vi "Basic Example.vi"() -> ()   [LabVIEW 2014]
uses:
  <userlib>/_NI SPI IP/FPGA/Controllers/Public/Transfer Settings.ctl
  vi.lib/SPIAPI/Controls/SPI Settings.ctl
  vi.lib/SPIAPI/Controls/Signal Properties.ctl
  <vilib>/rvi/Emulation/niFpgaGetClockAttributes.vi
  <vilib>/rvi/Emulation/niFpgaSctlEmulationGetInTimedLoop.vi
  <vilib>/rvi/Emulation/niFpgaEmulationReportErrorSimple.vi
  <vilib>/rvi/interface/RandomDataEmulation/niFpgaRandomDataHandleErrors.vi
  <vilib>/rvi/Emulation/niFpgaCriticalErrorInLSC.vi
  <vilib>/rvi/DataTransferAndStorage/Container/XNode/niFpgaContainer.xnode
  <vilib>/rvi/interface/RandomDataEmulation/nirviRandomDataFpgaReadWriteTemplate.vi
  <userlib>/_NI SPI IP/FPGA/Controllers/NI SPI IP FPGA.lvlib
panel:
  in  "data rate (S/s)":u32=10000
  in  "Chip Select":u8
  in  "SPI Command":u64
  in  "SPI PHY Settings":T1 {"Direction Change Bit" max=64 step=1; "Transfer Length (bits)" min=1 max=64 step=1}
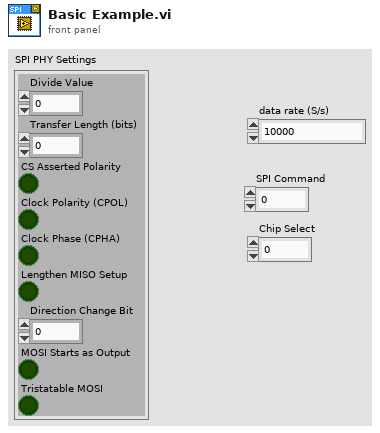
[diagram p1: front panel]
types:
  T1 = typedef "NI SPI IP FPGA.lvlib/Transfer Settings.ctl" = cluster{"Divide Value":u8, "Transfer Length (bits)":u8, "CS Asserted Polarity":bool, "Clock Polarity (CPOL)":bool, "Clock Phase (CPHA)":bool, "Lengthen MISO Setup":bool, "Direction Change Bit":u8, "MOSI Starts as Output":bool, "Tristatable MOSI":bool}
  T2 = typedef "SPI Settings.ctl" = cluster{"SCLK":T3, "Signal Settings":cluster{"MISO":refnum<k21>, "Signal_Enable":refnum<k21>, "Output?":bool}, "MOSI":T3, "CS0":T3, "CS1":T3, "CS2":T3, "CS3":T3, "CS4":T3, "CS5":T3}
  T3 = typedef "Signal Properties.ctl" = cluster{"Signal":refnum<k21>, "Signal_Enable":refnum<k21>, "Output?":bool}
  T4 = typedef "All SPI Settings.ctl" = cluster{"SPI Signal Settings":T2, "SPI Internal Signals":T5, "SPI PHY Settings":T1, "SPI Engine Source":refnum<k21>}
  T5 = typedef "Internal Data (SPI API).ctl" = cluster{"DLU To SPI Engine Data FIFO":refnum<k21>, "SPI Engine to DLU Data FIFO":refnum<k21>, "Data to SPI Engine (Cache) Register":refnum<k21>, "SPI PHY Settings to SPI Engine (Cahche) Register":refnum<k21>}
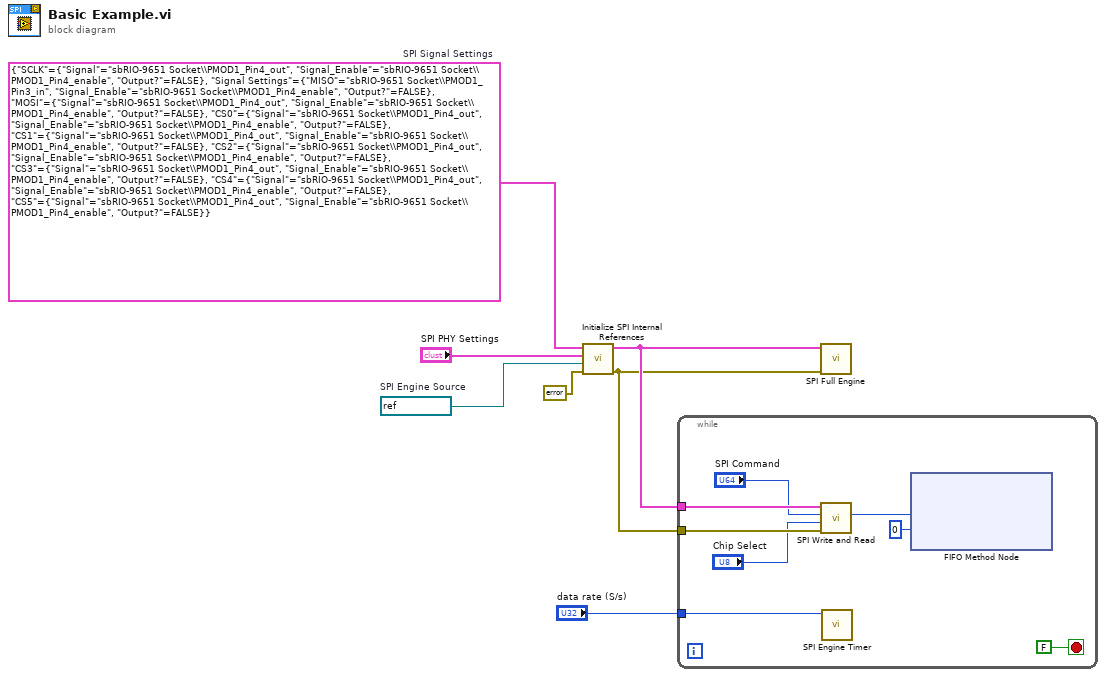
[diagram p0: block diagram]
diagram:
  w7 = T2 {"SCLK"={"Signal"="sbRIO-9651 Socket\\PMOD1_Pin4_out", "Signal_Enable"="sbRIO-9651 Socket\\PMOD1_Pin4_enable", "Output?"=FALSE}, "Signal Settings"={"MISO"="sbRIO-9651 Socket\\PMOD1_Pin3_in", "Signal_Enable"="sbRIO-9651 Socket\\PMOD1_Pin4_enable", "Output?"=FALSE}, "MOSI"={"Signal"="sbRIO-9651 Socket\\PMOD1_Pin4_out", "Signal_Enable"="sbRIO-9651 Socket\\PMOD1_Pin4_enable", "Output?"=FALSE}, "CS0"={"Signal"="sbRIO-9651 Socket\\PMOD1_Pin4_out", "Signal_Enable"="sbRIO-9651 Socket\\PMOD1_Pin4_enable", "Output?"=FALSE}, "CS1"={"Signal"="sbRIO-9651 Socket\\PMOD1_Pin4_out", "Signal_Enable"="sbRIO-9651 Socket\\PMOD1_Pin4_enable", "Output?"=FALSE}, "CS2"={"Signal"="sbRIO-9651 Socket\\PMOD1_Pin4_out", "Signal_Enable"="sbRIO-9651 Socket\\PMOD1_Pin4_enable", "Output?"=FALSE}, "CS3"={"Signal"="sbRIO-9651 Socket\\PMOD1_Pin4_out", "Signal_Enable"="sbRIO-9651 Socket\\PMOD1_Pin4_enable", "Output?"=FALSE}, "CS4"={"Signal"="sbRIO-9651 Socket\\PMOD1_Pin4_out", "Signal_Enable"="sbRIO-9651 Socket\\PMOD1_Pin4_enable", "Output?"=FALSE}, "CS5"={"Signal"="sbRIO-9651 Socket\\PMOD1_Pin4_out", "Signal_Enable"="sbRIO-9651 Socket\\PMOD1_Pin4_enable", "Output?"=FALSE}}  # SPI Signal Settings
  w5 = refnum<k21> "120MHz"  # SPI Engine Source
  n1 = call "Initialize SPI Internal References.vi"("error in"=errorcluster {"status"=FALSE, "code"=0, "source"=""}, "SPI Engine Source"=w5, "SPI PHY Settings"="SPI PHY Settings", "SPI Signal Settings"=w7) -> ("error out"=w2:errorcluster, "SPI Engine Reference"=w3:T4)  [unwired: 6 in]
  n2 = while {
    tunnel: w3 -> [w15]
    tunnel: w2 -> [w14]
    tunnel: "data rate (S/s)" -> [w8]
    stop <- FALSE stop-if-true
    n3 = call "SPI Write and Read.vi"("error in (no error)"=w14, "Chip Select"="Chip Select", "SPI Command"="SPI Command", "All SPI Settings"=w15) -> ("SPI Return Data"=w10:u64)  [unwired: 4 in, 3 out]
    n4 = call "SPI Engine Timer.vi"("data rate (S/s)"=w8) -> ()  [unwired: 10 in, 1 out]
    n5 = xnode ("FIFO Method Node")("Element"=w10, "Timeout"=0) -> ()  [unwired: 1 in, 2 out]
  }
  n6 = call "SPI Full Engine.vi"("error in (no error)"=w2, "All SPI Settings"=w3) -> ()  [unwired: 10 in]
